vi "Configuration reader.vi"(0 "refnum":T1, 5 "error in (no error)":errorcluster) -> (1 "Velocity":dbl, 2 "X offset":i32=693 step=1, 3 "Y travel":dbl min=0.0 max=5.0 step=0.0001, 4 "X travel":dbl min=0.0 max=50.0 step=0.0001, 6 "Y offset":i32=406 step=1, 7 "Acceleration":dbl, 8 "Width (px)":i32=240, 9 "Speed (µm/s)":i32=1000, 10 "XPS_Address":string, 11 "Axis 1 group":i32, 12 "Precision (%)":dbl=1.0 min=1.0 max=100.0 step=1.0 format="%#_3g", 13 "Pixel size":dbl=12.19 step=0.01, 14 "Heigth (px)":i32=240, 15 "Laser Com Delay":i32, 16 "Height  step \ndivider":i32=2, 17 "VISA Laser port":string, 18 "Axis 2 group":i32, 19 "error out":errorcluster)   [LabVIEW 2016]
uses:
  <vilib>/Utility/config.llb/Config Data RefNum.ctl
  <vilib>/Utility/config.llb/Read Key (I32).vi
  <vilib>/Utility/config.llb/Read Key (Double).vi
  <vilib>/Utility/config.llb/Read Key (String).vi
  <vilib>/Utility/config.llb/NI_LVConfig.lvlib
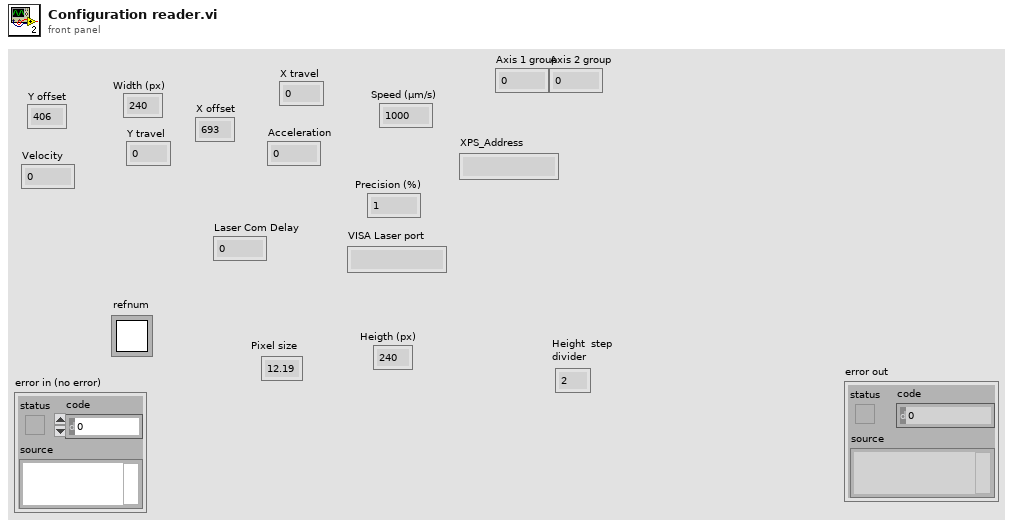
[diagram p1: front panel]
types:
  T1 = typedef "NI_LVConfig.lvlib/Config Data RefNum.ctl" = refnum<k1>
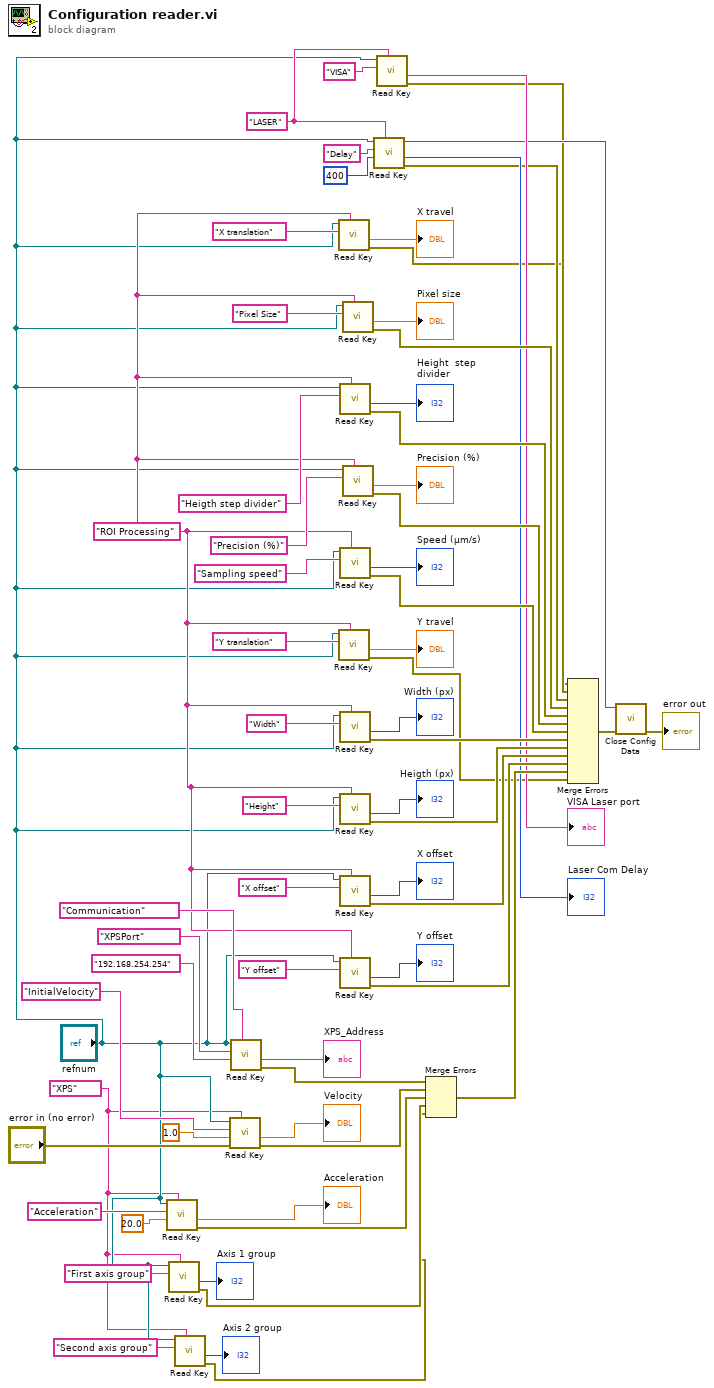
[diagram p0: block diagram]
diagram:
  w18 = "LASER" ("section")
  w34 = "ROI Processing" ("section")
  w9 = "XPS" ("section")
  n1 = call-poly <vilib>:"Read Key.vi"("section"=w9, "default value"=20.0, "key"="Acceleration", "refnum"="refnum") -> ("error out"=w35:errorcluster, "value"=→"Acceleration":dbl)  [unwired: 4 in, 2 out]
  n2 = call-poly <vilib>:"Read Key.vi"("section"=w9, "key"="First axis group", "refnum"="refnum") -> ("error out"=w4:errorcluster, "value"=→"Axis 1 group":i32)  [unwired: 5 in, 2 out]
  n3 = call-poly <vilib>:"Read Key.vi"("section"=w9, "key"="Second axis group", "refnum"="refnum") -> ("error out"=w3:errorcluster, "value"=→"Axis 2 group":i32)  [unwired: 5 in, 2 out]
  n4 = call-poly <vilib>:"Read Key.vi"("section"=w9, "error in (no error)"="error in (no error)", "default value"=1.0, "key"="InitialVelocity", "refnum"="refnum") -> ("error out"=w36:errorcluster, "value"=→"Velocity":dbl)  [unwired: 3 in, 2 out]
  n5 = call-poly <vilib>:"Read Key.vi"("section"="Communication", "default value"="192.168.254.254", "key"="XPSPort", "refnum"="refnum") -> ("error out"=w37:errorcluster, "value"=→"XPS_Address":string)  [unwired: 4 in, 2 out]
  n6 = call-poly <vilib>:"Read Key.vi"("section"=w34, "key"="X translation", "refnum"="refnum") -> ("error out"=w1:errorcluster, "value"=→"X travel":dbl)  [unwired: 5 in, 2 out]
  n7 = call-poly <vilib>:"Read Key.vi"("section"=w34, "key"="Y translation", "refnum"="refnum") -> ("error out"=w2:errorcluster, "value"=→"Y travel":dbl)  [unwired: 5 in, 2 out]
  n8 = call-poly <vilib>:"Read Key.vi"("section"=w34, "key"="Heigth step divider", "refnum"="refnum") -> ("error out"=w46:errorcluster, "value"=→"Height  step \ndivider":i32)  [unwired: 5 in, 2 out]
  n9 = call-poly <vilib>:"Read Key.vi"("section"=w34, "key"="Sampling speed", "refnum"="refnum") -> ("error out"=w44:errorcluster, "value"=→"Speed (µm/s)":i32)  [unwired: 5 in, 2 out]
  n10 = call-poly <vilib>:"Read Key.vi"("section"=w34, "key"="Width", "refnum"="refnum") -> ("error out"=w43:errorcluster, "value"=→"Width (px)":i32)  [unwired: 5 in, 2 out]
  n11 = call-poly <vilib>:"Read Key.vi"("section"=w34, "key"="Height", "refnum"="refnum") -> ("error out"=w42:errorcluster, "value"=→"Heigth (px)":i32)  [unwired: 5 in, 2 out]
  n12 = call-poly <vilib>:"Read Key.vi"("section"=w34, "key"="X offset", "refnum"="refnum") -> ("error out"=w41:errorcluster, "value"=→"X offset":i32)  [unwired: 5 in, 2 out]
  n13 = call-poly <vilib>:"Read Key.vi"("section"=w34, "key"="Y offset", "refnum"="refnum") -> ("error out"=w40:errorcluster, "value"=→"Y offset":i32)  [unwired: 5 in, 2 out]
  n14 = call-poly <vilib>:"Read Key.vi"("section"=w34, "key"="Pixel Size", "refnum"="refnum") -> ("error out"=w47:errorcluster, "value"=→"Pixel size":dbl)  [unwired: 5 in, 2 out]
  n15 = call-poly <vilib>:"Read Key.vi"("section"=w34, "key"="Precision (%)", "refnum"="refnum") -> ("error out"=w45:errorcluster, "value"=→"Precision (%)":dbl)  [unwired: 5 in, 2 out]
  n16 = call-poly <vilib>:"Read Key.vi"("section"=w18, "default value"=400, "key"="Delay", "refnum"="refnum") -> ("error out"=w12:errorcluster, "value"=→"Laser Com Delay":i32, "refnum out"=w13:T1)  [unwired: 4 in, 1 out]
  n17 = call-poly <vilib>:"Read Key.vi"("section"=w18, "key"="VISA", "refnum"="refnum") -> ("error out"=w11:errorcluster, "value"=→"VISA Laser port":string)  [unwired: 5 in, 2 out]
  n18 = Merge Errors(w37, w36, w35, w4, w3) -> (w38:errorcluster)
  n19 = Merge Errors(w1, w11, w12, w47, w46, w45, w44, w43, w42, w41, w40, w38, w2) -> (w39:errorcluster)
  n20 = call <vilib>:"Close Config Data.vi"("error in (no error)"=w39, "refnum"=w13) -> ("error out"=→"error out":errorcluster)  [unwired: 8 in, 1 out]
